vi "Teardown.vi"(8 "error in (no error)":errorcluster, 11 "LUnit Test Commands In":refnum<class "Test Commands.lvclass">) -> (0 "error out":errorcluster, 3 "LUnit Test Commands Out":refnum<class "Test Commands.lvclass">)   [LabVIEW 2019, in "Test Commands.lvclass"]
doc: "Teardown method called by the testing framework to tear down test fixture after each test method is called."
uses:
  Test Commands.lvclass
  Test Commands.lvclass/Test Commands.ctl
  <vilib>/Astemes/LUnit/Test Case.lvclass
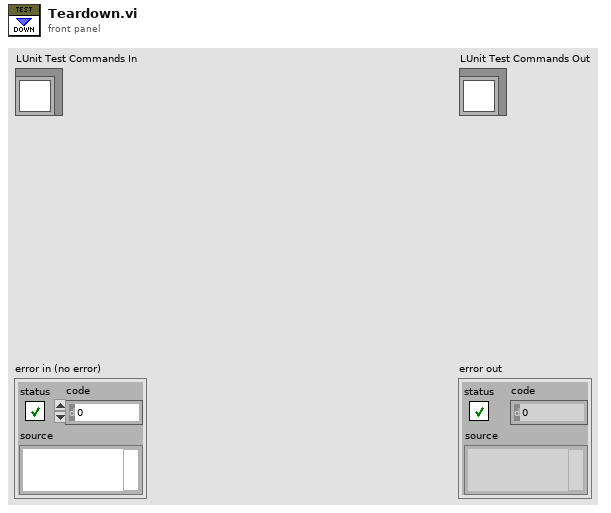
[diagram p1: front panel]
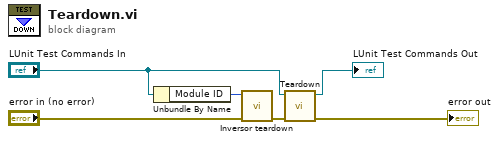
[diagram p0: block diagram]
diagram:
  n1 = Unbundle By Name("LUnit Test Commands In") -> ("Module ID"=w1:i32)
  n2 = call "Inversor teardown.vi"("error in"="error in (no error)", "Module ID"=w1) -> ("error out"=w3:errorcluster)  [unwired: 9 in]
  n3 = call-parent "Teardown.vi"("error in (no error)"=w3, "LUnit Test Case In"="LUnit Test Commands In") -> ("error out"=→"error out":errorcluster, "LUnit Test Case Out"=→"LUnit Test Commands Out":refnum<class "Test Commands.lvclass">)  [unwired: 8 in]
